vi "dataFifoUpdate.vi"(5 "Data Notifier":refnum<notifier>, 7 "clustPointagFin":T1, 9 "Data Queue":refnum<queue>, 11 "error in (no error)":errorcluster) -> (15 "error out":errorcluster)   [LabVIEW 2020, in "Acquisition.lvlib"]
doc: "Perform the acquisition. Replace the contents of this diagram with calls to acquisition hardware."
uses:
  Acquisition.lvlib
  SETTING/data_Queue.ctl
  SETTING/data_Display.ctl
  SETTING/clustOA.ctl
  <vilib>/Analysis/Matrix/Datatypes/RealMatrix.ctl
  <vilib>/Analysis/Matrix/NI_Matrix.lvlib
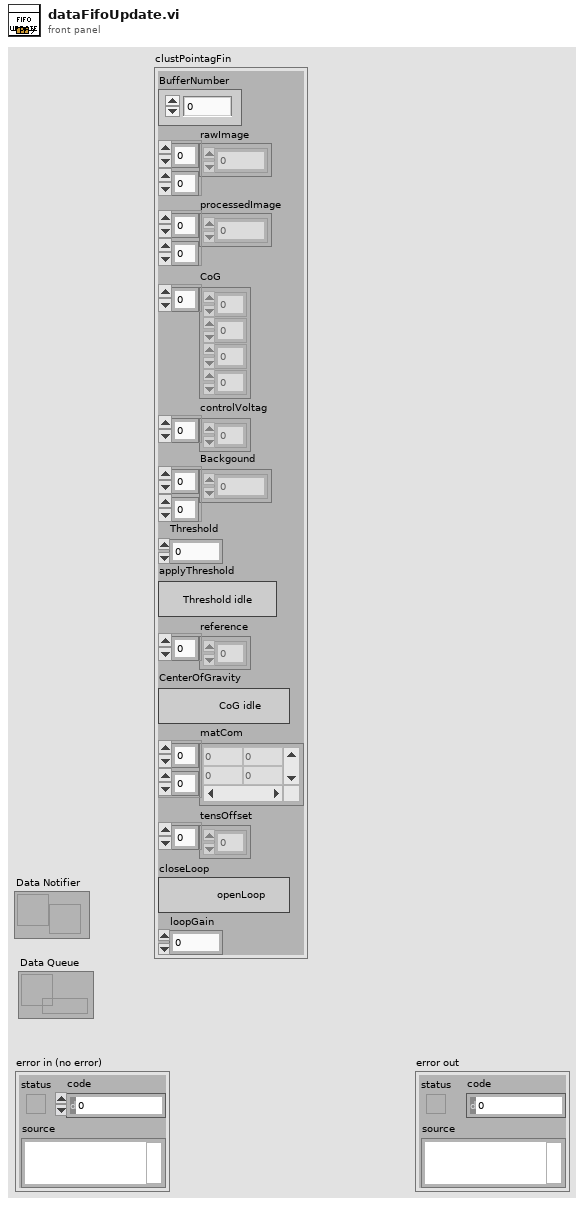
[diagram p1: front panel]
types:
  T1 = typedef "clustOA.ctl" = cluster{"BufferNumber":u32, "rawImage":u16[][], "processedImage":sgl[][], "CoG":dbl[], "controlVoltag":dbl[], "Backgound":sgl[][], "Threshold":dbl, "applyThreshold":bool, "reference":dbl[], "CenterOfGravity":bool, "matCom":T2, "tensOffset":dbl[], "closeLoop":bool, "loopGain":dbl}
  T2 = typedef "NI_Matrix.lvlib/RealMatrix.ctl" = dbl[][]
  T3 = typedef "data_Queue.ctl" = cluster{"tabIma":u16[][], "tabCdG":sgl[], "vectCom":sgl[]}
  T4 = typedef "data_Display.ctl" = cluster{"tabIma":sgl[][], "tabCdG":sgl[], "vectCom":sgl[]}
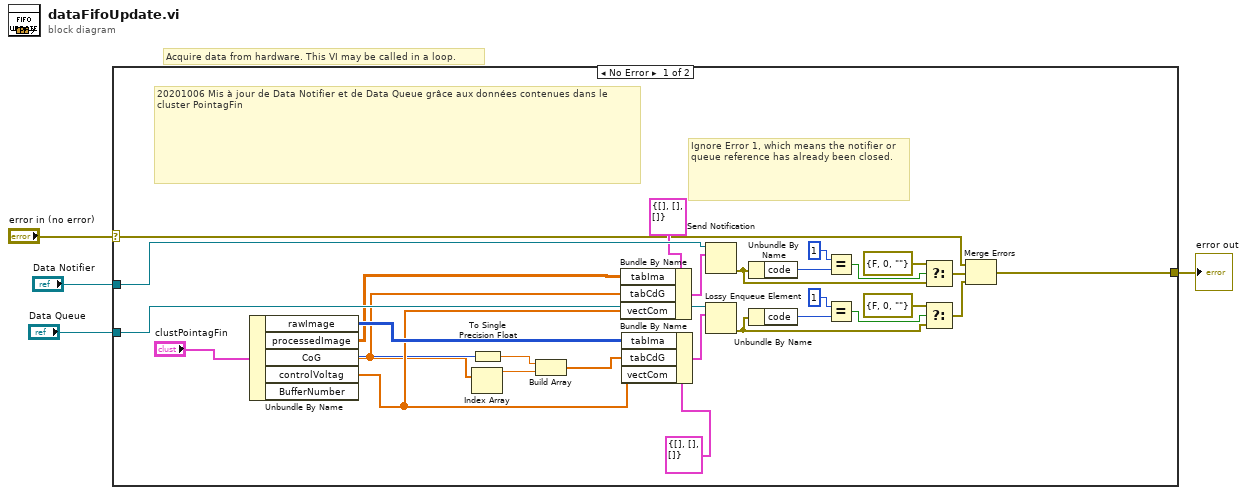
[diagram p0: block diagram]
diagram:
  # "Acquire data from hardware. This VI may be called in a loop."
  n1 = case shown="No Error" "error in (no error)" {
    selector: "error in (no error)" -> [w13 w34]
    tunnel: [w33 w34] -> w3
    tunnel: "Data Notifier" -> [w32 _]
    tunnel: "Data Queue" -> [w19 _]
    frame No Error {
      # "Ignore Error 1, which means the notifier or queue reference has already been closed."
      # "20201006 Mis à jour de Data Notifier et de Data Queue grâce aux données contenues dans le cluster PointagFin"
      n2 = Unbundle By Name("clustPointagFin") -> ("rawImage"=w12:u16[][], "processedImage"=w11:sgl[][], "CoG"=w6:dbl[], "controlVoltag"=w10:dbl[], "BufferNumber"=w9:u32)
      n3 = Index Array(array=w6) -> (element=w5:dbl)  [unwired: 1 in]
      n4 = To Single Precision Float(number=w9) -> (single precision float=w7:sgl)
      n5 = Build Array(w7, w5) -> (w8:dbl[])
      n6 = Bundle By Name(cluster=T4 {"tabIma"=[], "tabCdG"=[], "vectCom"=[]} ("data2Display"), "tabIma"=w11, "tabCdG"=w6, "vectCom"=w10) -> (w17:T4)
      n7 = Bundle By Name(cluster=T3 {"tabIma"=[], "tabCdG"=[], "vectCom"=[]} ("Cluster"), "tabIma"=w12, "tabCdG"=w8, "vectCom"=w10) -> (w15:T3)
      n8 = Send Notification(notification=w17, notifier=w32) -> (error out=w28:errorcluster)  [unwired: 1 in, 1 out]
      n9 = Lossy Enqueue Element(queue=w19, element=w15) -> (error out=w24:errorcluster)  [unwired: 1 in, 3 out]
      n10 = Unbundle By Name(w28) -> ("code"=w31:i32)
      n11 = Unbundle By Name(w24) -> ("code"=w21:i32)
      n12 = Equal?(x=1, y=w31) -> (x = y?=w29:bool)
      n13 = Equal?(x=1, y=w21) -> (x = y?=w23:bool)
      n14 = Select(t=errorcluster {"status"=FALSE, "code"=0, "source"=""} ("error constant"), s=w29, f=w28) -> (s? t:f=w27:errorcluster)
      n15 = Select(t=errorcluster {"status"=FALSE, "code"=0, "source"=""} ("error constant"), s=w23, f=w24) -> (s? t:f=w20:errorcluster)
      n16 = Merge Errors(w13, w27, w20) -> (w33:errorcluster)
    }
    frame Error {
    }
  }
  "error out" <- w3
